vi "cRIO ping.vi"(8 "Error in":errorcluster, 10 "Ping Timeout (ms)":i32, 11 "IP Address":string) -> (0 "Ping error out":errorcluster, 3 "Ping Response":string)   [LabVIEW 2016, in "Top Level.lvlib"]
doc: "Pings IP address and returns response"
uses:
  top level/Top Level.lvlib
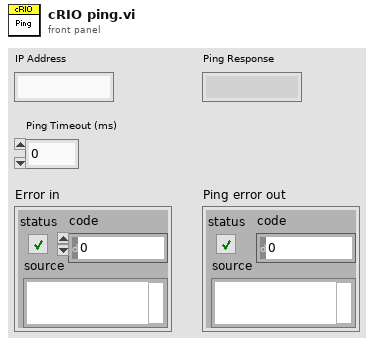
[diagram p1: front panel]
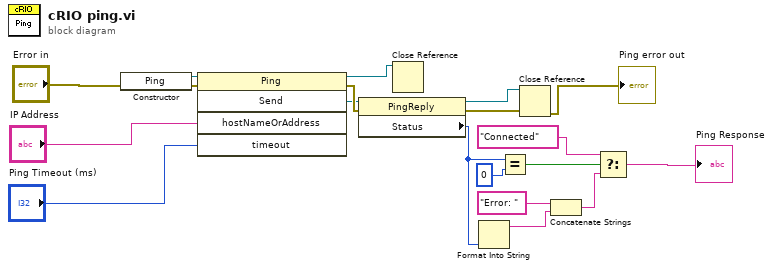
[diagram p0: block diagram]
diagram:
  n1 = constructor class="Ping"(error in="Error in") -> (reference out=w3:refnum<k24>, error out=w6:errorcluster)  [unwired: 2 in, 1 out]
  n2 = invoke class="Ping" method="Send"(reference=w3, error in=w6, "hostNameOrAddress"="IP Address", "timeout"="Ping Timeout (ms)") -> (reference out=w11:refnum<k24>, error out=w10:errorcluster, "Send"=w2:refnum<k24>)  [unwired: 1 in, 2 out]
  n3 = property class="PingReply"(reference=w2, error in=w10) -> (reference out=w4:refnum<k24>, error out=w8:errorcluster, "Status"=w16:i32)
  n4 = Close Reference(reference=w11) -> ()  [unwired: 1 in, 1 out]
  n5 = Format Into String(w16) -> (resulting string=w19:string)  [unwired: 3 in, 1 out]
  n6 = Equal?(x=w16, y=0) -> (x = y?=w13:bool)
  n7 = Close Reference(reference=w4, error in (no error)=w8) -> (error out=→"Ping error out":errorcluster)
  n8 = Concatenate Strings("Error: ", w19) -> (w17:string)
  n9 = Select(t="Connected", s=w13, f=w17) -> (s? t:f=→"Ping Response":string)
